vi "FTW-Test-JSON-ObjectJoin.vi"() -> (0 "Test Result":errorcluster)   [LabVIEW 2014]
uses:
  src/json/FTW-JSON-UpdateMode.ctl
  src/error/FTW-ERR-ThrowInfo.vi
  src/error/FTW-ERR-ThrowError.vi
  src/error/FTW-ERR-CallChain.vi
  src/string/FTW-STR-ReplaceWhitespace.vi
panel:
  out "Joined Objects":string[](array[string])
  out "JSON to Join":string
  out "Original JSON":string
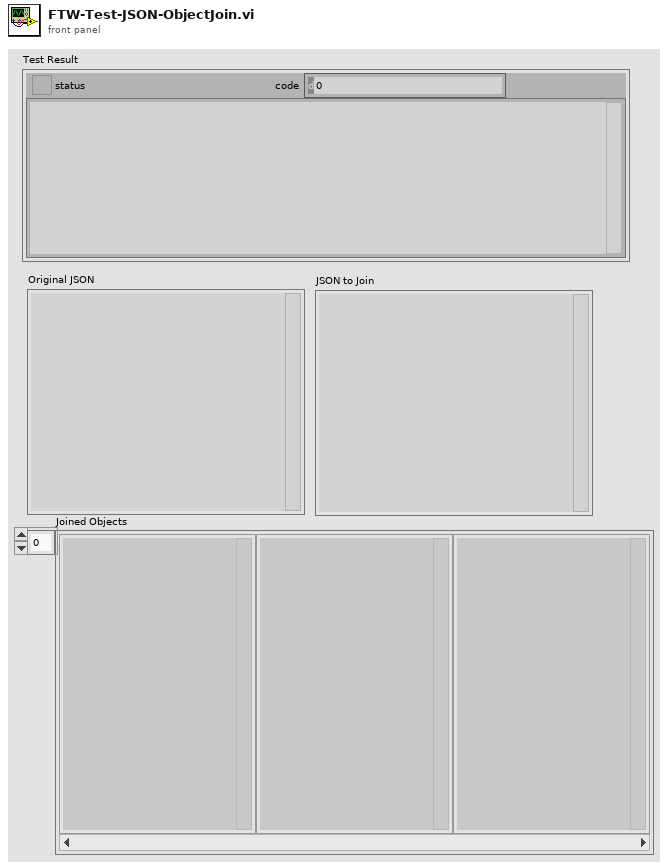
[diagram p1: front panel]
types:
  T1 = typedef "FTW-JSON-UpdateMode.ctl" = enum32{"Upsert", "Update Only", "Insert Only"}
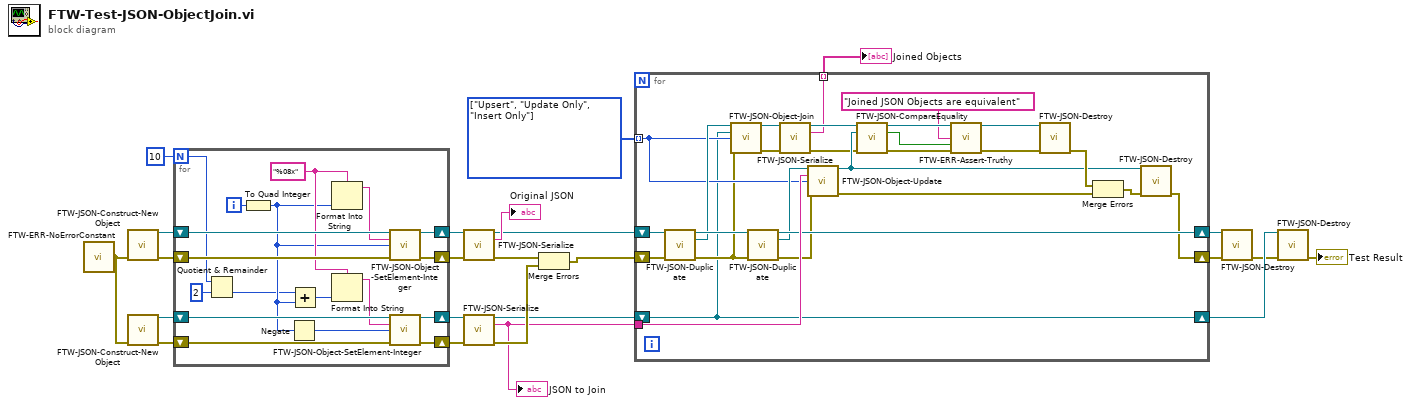
[diagram p0: block diagram]
diagram:
  w9 = T1[] [enum."Upsert", enum."Update Only", enum."Insert Only"] items=["Upsert", "Update Only", "Insert Only"]
  n1 = call "FTW-ERR-NoErrorConstant.vi"() -> ("no error"=w18:errorcluster)
  n2 = call "FTW-JSON-Construct-NewObject.vi"("error in"=w18) -> ("JSON Object"=w20:refnum<data-value>, "error out"=w19:errorcluster)  [unwired: 13 in]
  n3 = call "FTW-JSON-Construct-NewObject.vi"("error in"=w18) -> ("JSON Object"=w16:refnum<data-value>, "error out"=w17:errorcluster)  [unwired: 13 in]
  n4 = for {
    N: 10 -> [w27]
    shift-right: [w38] -> w22
    shift-left: w19 -> [w40]
    shift-right: [w41] -> w23
    shift-left: w20 -> [w42]
    shift-right: [w33] -> w14
    shift-left: w17 -> [w35]
    shift-right: [w34] -> w15
    shift-left: w16 -> [w36]
    i -> [w37]
    w32 = "%08x" ("format string")
    n5 = Quotient & Remainder(x=w27, y=2) -> (floor(x/y)=w25:i32)  [unwired: 1 out]
    n6 = To Quad Integer(1:w37) -> (0:w29:i64)
    n7 = Negate(x=w29) -> (-x=w30:i64)
    n8 = Add(x=w25, y=w29) -> (x+y=w28:i64)
    n9 = Format Into String(format string=w32, w29) -> (resulting string=w39:string)  [unwired: 2 in, 1 out]
    n10 = Format Into String(format string=w32, w28) -> (resulting string=w31:string)  [unwired: 2 in, 1 out]
    n11 = call "FTW-JSON-Object-SetElement-Integer.vi"("JSON Object"=w42, "Key"=w39, "Value"=w29, "error in"=w40) -> ("JSON Object out"=w41:refnum<data-value>, "error out"=w38:errorcluster)  [unwired: 10 in]
    n12 = call "FTW-JSON-Object-SetElement-Integer.vi"("JSON Object"=w36, "Key"=w31, "Value"=w30, "error in"=w35) -> ("JSON Object out"=w34:refnum<data-value>, "error out"=w33:errorcluster)  [unwired: 10 in]
  }
  n13 = call "FTW-JSON-Serialize.vi"("JSON Object"=w23, "error in"=w22) -> ("JSON Object out"=w13:refnum<data-value>, "JSON String (UTF-8)"=→"Original JSON":string, "error out"=w11:errorcluster)  [unwired: 11 in]
  n14 = call "FTW-JSON-Serialize.vi"("JSON Object"=w15, "error in"=w14) -> ("JSON Object out"=w8:refnum<data-value>, "JSON String (UTF-8)"=w7:string, "error out"=w12:errorcluster)  [unwired: 11 in]
  "JSON to Join" <- w7
  n15 = Merge Errors(w11, w12) -> (w10:errorcluster)
  n16 = for {
    tunnel: w9 -> [w57] mode=indexing
    tunnel: w7 -> [w65]
    shift-right: [w63] -> w6
    shift-left: w13 -> [w68]
    shift-right: [w60] -> w5
    shift-left: w10 -> [w66]
    tunnel: [w52] -> w4 mode=indexing
    shift-right: [w43] -> w3
    shift-left: w8 -> [w43]
    n17 = call "FTW-JSON-Duplicate.vi"("JSON Object"=w68, "error in"=w66) -> ("JSON Object out"=w67:refnum<data-value>, "Duplicated JSON Object"=w59:refnum<data-value>, "error out"=w50:errorcluster)  [unwired: 11 in]
    n18 = call "FTW-JSON-Object-Join.vi"("JSON Object"=w59, "JSON Object to Merge"=w43, "Join Mode"=w57, "error in"=w50) -> ("JSON Object out"=w55:refnum<data-value>, "error out"=w51:errorcluster)  [unwired: 10 in]
    n19 = call "FTW-JSON-Duplicate.vi"("JSON Object"=w67, "error in"=w50) -> ("JSON Object out"=w63:refnum<data-value>, "Duplicated JSON Object"=w58:refnum<data-value>, "error out"=w56:errorcluster)  [unwired: 11 in]
    n20 = call "FTW-JSON-Serialize.vi"("JSON Object"=w55, "error in"=w51) -> ("JSON Object out"=w54:refnum<data-value>, "JSON String (UTF-8)"=w52:string, "error out"=w48:errorcluster)  [unwired: 11 in]
    n21 = call "FTW-JSON-Object-Update.vi"("JSON Object"=w58, "JSON Object to Merge"=w65, "Update Mode"=w57, "error in"=w56) -> ("JSON Object out"=w53:refnum<data-value>, "error out"=w49:errorcluster)  [unwired: 10 in]
    n22 = call "FTW-JSON-CompareEquality.vi"("JSON Object"=w54, "JSON Object to Compare"=w53, "error in"=w48) -> ("JSON Object out"=w64:refnum<data-value>, "Equal?"=w45:bool, "error out"=w47:errorcluster)  [unwired: 10 in]
    n23 = call "FTW-ERR-Assert-Truthy.vi"("Assertion"="Joined JSON Objects are equivalent", "Assertion holds true?"=w45, "error in"=w47) -> ("error out"=w46:errorcluster)  [unwired: 12 in]
    n24 = call "FTW-JSON-Destroy.vi"("JSON Object"=w64, "error in"=w46) -> ("error out"=w62:errorcluster)  [unwired: 13 in]
    n25 = Merge Errors(w62, w49) -> (w61:errorcluster)
    n26 = call "FTW-JSON-Destroy.vi"("JSON Object"=w53, "error in"=w61) -> ("error out"=w60:errorcluster)  [unwired: 13 in]
  }
  "Joined Objects" <- w4
  n27 = call "FTW-JSON-Destroy.vi"("JSON Object"=w6, "error in"=w5) -> ("error out"=w2:errorcluster)  [unwired: 13 in]
  n28 = call "FTW-JSON-Destroy.vi"("JSON Object"=w3, "error in"=w2) -> ("error out"=→"Test Result":errorcluster)  [unwired: 13 in]
